vi "Build Path Root.vi"(8 "error in":errorcluster, 11 "Report Generator in":refnum<class "Report Generator.lvclass">) -> (0 "error out":errorcluster, 3 "Report Generator out":refnum<class "Report Generator.lvclass">)   [LabVIEW 2018, in "Report Generator.lvlib" / "Report Generator.lvclass"]
uses:
  Report Generator.lvclass
  Report Generator.lvclass/Report Generator.ctl
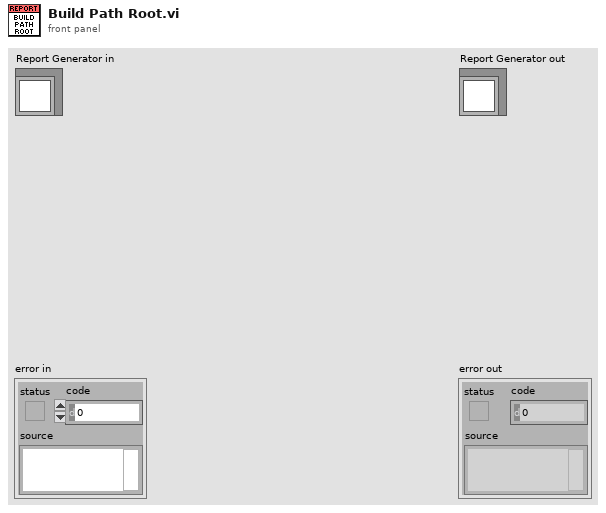
[diagram p1: front panel]
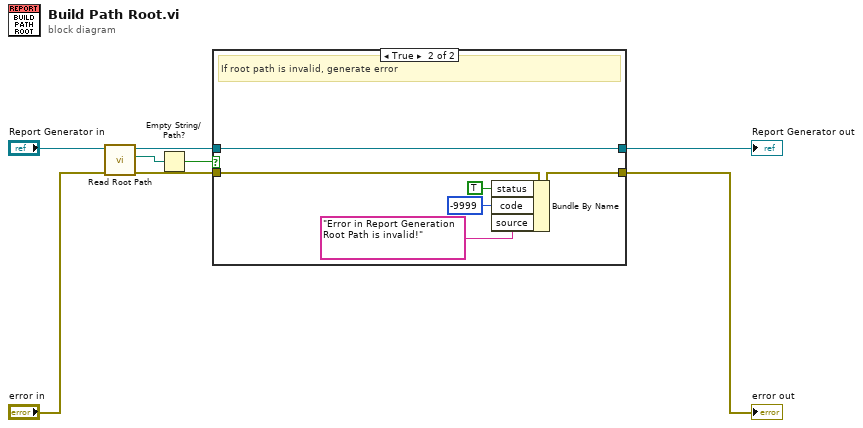
[diagram p0: block diagram]
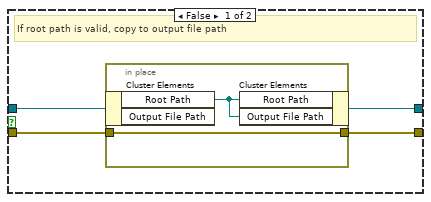
[diagram p2: hidden frame]
diagram:
  n1 = call "Read Root Path.vi"("error in (no error)"="error in", "Report Generator in"="Report Generator in") -> ("error out"=w3:errorcluster, "Root Path"=w6:path, "Report Generator out"=w4:refnum<class "Report Generator.lvclass">)  [unwired: 7 in]
  n2 = Empty String/Path?(string/path=w6) -> (empty?=w5:bool)
  n3 = case shown="True" w5 {
    tunnel: w4 -> [w12 w20]
    tunnel: w3 -> [w10 w19]
    tunnel: [w11 w20] -> w2
    tunnel: [w9 w18] -> w1
    frame False {
      # "If root path is valid, copy to output file path"
      n4 = in-place {
        in-place-border: w10 -> [w14]
        in-place-border: [w14] -> w9
        n5 = in-place-cluster #1(w12) -> ("Root Path"=w13:path)  [unwired: 1 out]
        n6 = in-place-cluster #1("Root Path"=w13, "Output File Path"=w13) -> (w11:refnum<class "Report Generator.lvclass">)
      }
    }
    frame True {
      # "If root path is invalid, generate error"
      n7 = Bundle By Name(cluster=w19, "status"=TRUE, "code"=-9999, "source"="Error in Report Generation Root Path is invalid!") -> (w18:errorcluster)
    }
  }
  "error out" <- w1
  "Report Generator out" <- w2
